vi "！所有实验仪器主函数必须添加此代码！！！.vi"   [LabVIEW 2014]
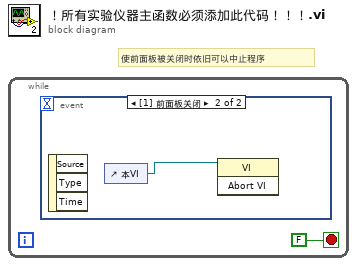
[diagram p0: block diagram]
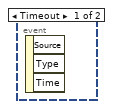
[diagram p2: hidden frame]
diagram:
  # "使前面板被关闭时依旧可以中止程序"
  n1 = while {
    stop <- FALSE stop-if-true
    n2 = event shown="[1] 前面板关闭" {
      selector: _ -> [_ _]
      dyn-events: _ -> [_ _]
      timeout: _ -> [_ _]
      event Timeout {
        n3 = event-data() -> ()  [unwired: 1 in, 3 out]
      }
      event Panel Close {
        n4 = event-data() -> ()  [unwired: 1 in, 3 out]
        n5 = control-ref of="本VI"() -> (w2:refnum<vi>)
        n6 = invoke class="VI" method="Abort VI"(reference=w2) -> ()  [unwired: 2 in, 3 out]
      }
    }
  }
